vi "Auto_Routine_DepositConeBalance.vi"(8 "error in (no error)":errorcluster) -> (0 "error out":errorcluster)   [LabVIEW 2020]
doc: "deposits cone, drives backwards, balances. Starts from 3rd node from non pickup edge\n\ninputs:\n--ErrorIn--\noutputs:\n--ErrorOut--"
uses:
  Arm/ArmGamePiecePreset.ctl
  Arm/ArmPositionPreset.ctl
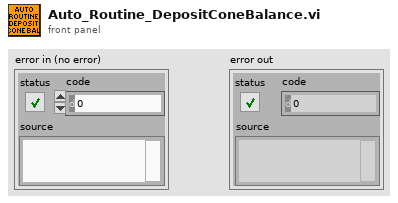
[diagram p1: front panel]
types:
  T1 = typedef "ArmGamePiecePreset.ctl" = enum16{"Cube", "Cone"}
  T2 = typedef "ArmPositionPreset.ctl" = enum16{"Upper", "Lower", "Middle", "Shelf", "Floor"}
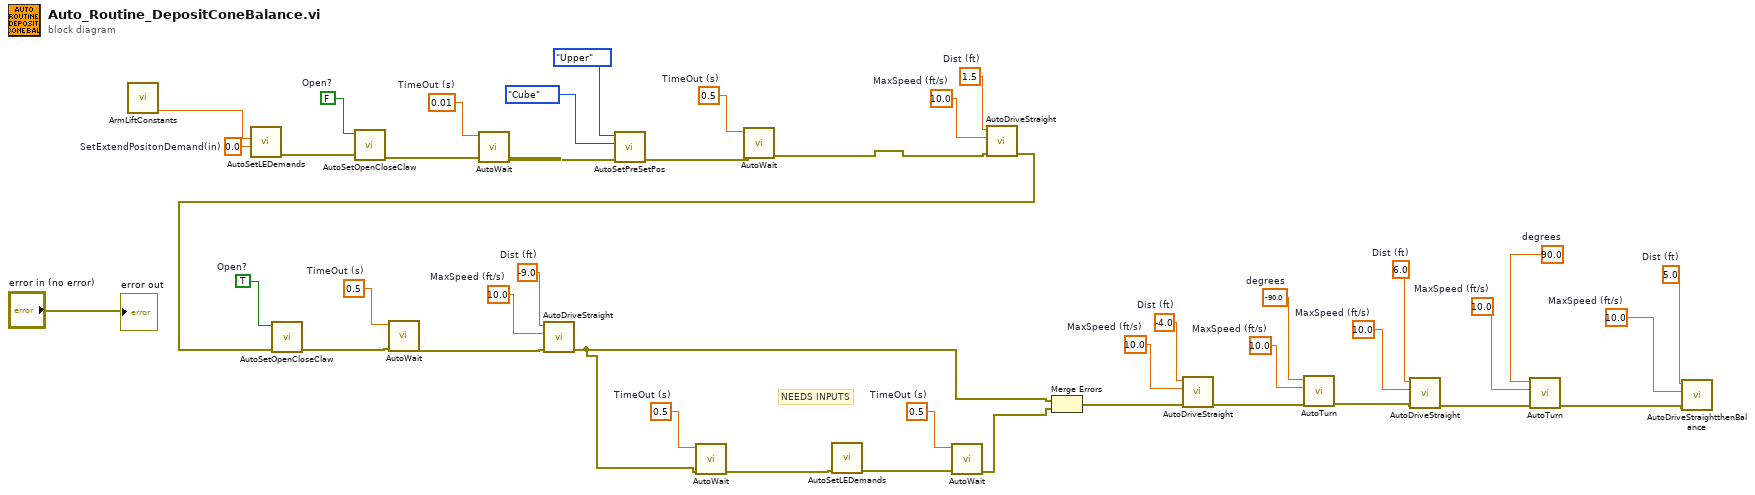
[diagram p0: block diagram]
diagram:
  w3 = 0.0  # SetExtendPositonDemand(in)
  w8 = 10.0  # MaxSpeed (ft/s)
  w9 = 5.0  # Dist (ft)
  w12 = 10.0  # MaxSpeed (ft/s)
  w13 = 90.0  # degrees
  w14 = 10.0  # MaxSpeed (ft/s)
  w15 = 6.0  # Dist (ft)
  w17 = 10.0  # MaxSpeed (ft/s)
  w18 = -90.0  # degrees
  w21 = -4.0  # Dist (ft)
  w22 = 10.0  # MaxSpeed (ft/s)
  w25 = 0.5  # TimeOut (s)
  w27 = 0.5  # TimeOut (s)
  w29 = -9.0  # Dist (ft)
  w30 = 10.0  # MaxSpeed (ft/s)
  w32 = 0.5  # TimeOut (s)
  w34 = TRUE  # Open?
  w35 = 1.5  # Dist (ft)
  w36 = 10.0  # MaxSpeed (ft/s)
  w38 = 0.5  # TimeOut (s)
  w40 = 0.01  # TimeOut (s)
  w42 = FALSE  # Open?
  # "NEEDS INPUTS"
  n1 = call "ArmLiftConstants.vi"() -> ("Starting Angle"=w2:dbl)  [unwired: 9 in, 2 out]
  n2 = call "AutoSetLEDemands.vi"("SetExtendPositonDemand(in)"=w3, "SetLIftPostionDemand(d)"=w2) -> ("error out"=w1:errorcluster)  [unwired: 9 in]
  n3 = call "AutoSetOpenCloseClaw.vi"("error in (no error)"=w1, "Open?"=w42) -> ("error out"=w41:errorcluster)  [unwired: 9 in]
  n4 = call "AutoWait.vi"("error in (no error)"=w41, "TimeOut (s)"=w40) -> ("error out"=w39:errorcluster)  [unwired: 9 in]
  n5 = call "AutoSetPreSetPos.vi"("error in (no error)"=w39, "Game Piece"=ArmGamePiecePreset."Cube", "Position"=ArmPositionPreset."Upper") -> ("error out"=w37:errorcluster)  [unwired: 8 in]
  n6 = call "AutoWait.vi"("error in (no error)"=w37, "TimeOut (s)"=w38) -> ("error out"=w4:errorcluster)  [unwired: 9 in]
  n7 = call "AutoDriveStraight.vi"("error in (no error)"=w4, "MaxSpeed (ft/s)"=w36, "Dist (ft)"=w35) -> ("error out"=w33:errorcluster)  [unwired: 8 in]
  n8 = call "AutoSetOpenCloseClaw.vi"("error in (no error)"=w33, "Open?"=w34) -> ("error out"=w31:errorcluster)  [unwired: 9 in]
  n9 = call "AutoWait.vi"("error in (no error)"=w31, "TimeOut (s)"=w32) -> ("error out"=w28:errorcluster)  [unwired: 9 in]
  n10 = call "AutoDriveStraight.vi"("error in (no error)"=w28, "MaxSpeed (ft/s)"=w30, "Dist (ft)"=w29) -> ("error out"=w5:errorcluster)  [unwired: 8 in]
  n11 = call "AutoWait.vi"("error in (no error)"=w5, "TimeOut (s)"=w27) -> ("error out"=w26:errorcluster)  [unwired: 9 in]
  n12 = call "AutoSetLEDemands.vi"("error in (no error)"=w26) -> ("error out"=w24:errorcluster)  [unwired: 10 in]
  n13 = call "AutoWait.vi"("error in (no error)"=w24, "TimeOut (s)"=w25) -> ("error out"=w23:errorcluster)  [unwired: 9 in]
  n14 = Merge Errors(w5, w23) -> (w20:errorcluster)
  n15 = call "AutoDriveStraight.vi"("error in (no error)"=w20, "MaxSpeed (ft/s)"=w22, "Dist (ft)"=w21) -> ("error out"=w19:errorcluster)  [unwired: 8 in]
  n16 = call "AutoTurn.vi"("error in (no error)"=w19, "MaxSpeed (ft/s)"=w17, "degrees"=w18) -> ("error out"=w16:errorcluster)  [unwired: 8 in]
  n17 = call "AutoDriveStraight.vi"("error in (no error)"=w16, "MaxSpeed (ft/s)"=w14, "Dist (ft)"=w15) -> ("error out"=w11:errorcluster)  [unwired: 8 in]
  n18 = call "AutoTurn.vi"("error in (no error)"=w11, "MaxSpeed (ft/s)"=w12, "degrees"=w13) -> ("error out"=w10:errorcluster)  [unwired: 8 in]
  n19 = call "AutoDriveStraightthenBalance.vi"("error in (no error)"=w10, "MaxSpeed (ft/s)"=w8, "Dist (ft)"=w9) -> ()  [unwired: 8 in, 1 out]
  "error out" <- "error in (no error)"
